vi "Read Measurement.vi"(8 "error in (no error)":errorcluster, 10 "Read Parameters":T1={"Channel (1: Channel 1)"=1, "Measurement Type (0: Frequency)"=0} {"Measurement Type (0: Frequency)" items=["Frequency", "Mean", "Period", "Pulse Duty", "Peak to Peak", "Cycle RMS", "Minimum", "Maximum", "Rise Time", "Fall Time", "Positive Width", "Negative Width", "Amplitude", "Cycle Mean", "High", "Low", "Negative Duty", "Positive Overshoot", "Negative Overshoot", "Cursor Mean", "Burst Width", "Positive Pulse Count", "Negative Pulse Count", "Rising Edge Count", "Falling Edge Count", "Area", "Cycle Area", "RMS", "Cursor RMS"]; "Channel (1: Channel 1)" items=["Channel 1"=1, "Channel 2"=2, "Channel 3"=3, "Channel 4"=4]}, 11 "EDUX1002G in":refnum<class "EDUX1002G.lvclass">) -> (0 "error out":errorcluster, 1 "Units":string, 2 "Measurement":dbl, 3 "EDUX1002G out":refnum<class "EDUX1002G.lvclass">)   [LabVIEW 2020, in "Osciloscope Tektronix.lvlib" / "EDUX1002G.lvclass"]
uses:
  EDUX1002G.lvclass
  C:/Users/Pablo/Osciloscope-Tek/TDS2000/Libraries/Osciloscope Tektronix/Clases/Osciloscope/Osciloscope.lvclass
  Osciloscope/Osciloscope.lvclass/Osciloscope.ctl
  Osciloscope/Read COM.vi
  <instrlib>/Agilent 2000 3000 X-Series/Public/Data/Read Measurement (Current Value).vi
  <instrlib>/Agilent 2000 3000 X-Series/Agilent 2000 3000 X-Series.lvlib
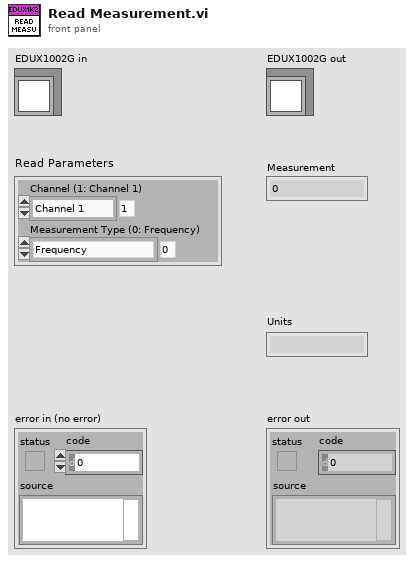
[diagram p1: front panel]
types:
  T1 = cluster{"Channel (1: Channel 1)":i32, "Measurement Type (0: Frequency)":i32}
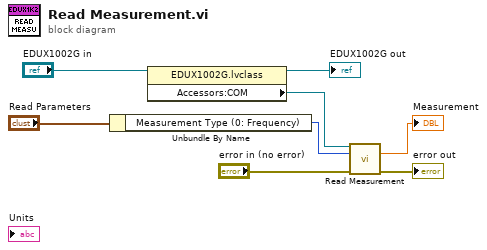
[diagram p0: block diagram]
diagram:
  n1 = Unbundle By Name("Read Parameters") -> ("Measurement Type (0: Frequency)"=w1:i32)
  n2 = property class="EDUX1002G.lvclass"(reference="EDUX1002G in") -> (reference out=→"EDUX1002G out":refnum<class "EDUX1002G.lvclass">, "Accessors:COM"=w4:refnum<visa-resource-name>)  [unwired: 1 in, 1 out]
  n3 = call-poly <instrlib>:"Read Measurement.vi"("VISA resource name"=w4, "Measurement Type (0: Peak-Peak)"=w1, "error in (no error)"="error in (no error)") -> ("Result Value"=→"Measurement":dbl, "error out"=→"error out":errorcluster)  [unwired: 10 in, 1 out]
